vi "Write Str Ref.vi"(8 "error in (no error)":errorcluster, 10 "Str Ref":refnum<vi>, 11 "Display Panel V3 in":refnum<class "Display Panel V3.lvclass">) -> (0 "error out":errorcluster, 3 "Display Panel V3 out":refnum<class "Display Panel V3.lvclass">)   [LabVIEW 2014, in "Display Panel.lvlib" / "Display Panel V3.lvclass"]
uses:
  Display Panel V3.lvclass
  Display Panel V3.lvclass/Display Panel V3.ctl
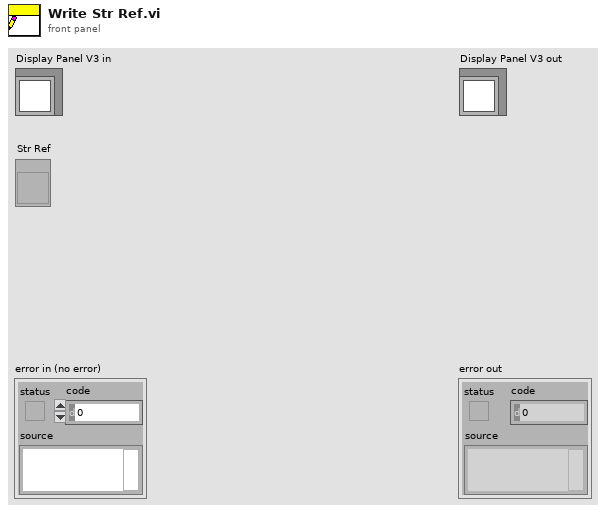
[diagram p1: front panel]
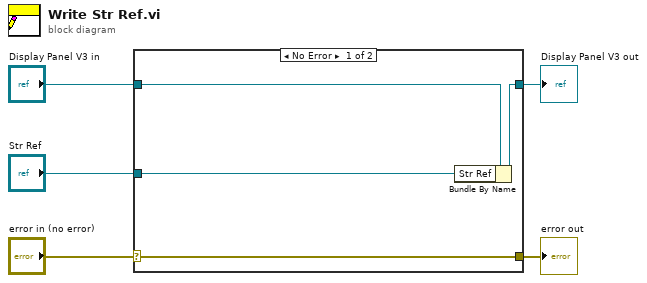
[diagram p0: block diagram]
diagram:
  n1 = case shown="No Error" "error in (no error)" {
    selector: "error in (no error)" -> [w9 w10]
    tunnel: [w9 w10] -> w4
    tunnel: [w7 w11] -> w2
    tunnel: "Display Panel V3 in" -> [w8 w11]
    tunnel: "Str Ref" -> [w6 _]
    frame No Error {
      n2 = Bundle By Name(cluster=w8, "Str Ref"=w6) -> (w7:refnum<class "Display Panel V3.lvclass">)
    }
    frame Error {
    }
  }
  "error out" <- w4
  "Display Panel V3 out" <- w2
